vi "subVI_Strain_Ass2.vi"() -> (0 "error out":errorcluster caption="에러 출력", 3 "data 2":waveform(dbl)[](array[waveform]) caption="Strain data")   [LabVIEW 2016]
uses:
  <vilib>/DAQmx/read.llb/DAQmx Read.vi
  <vilib>/DAQmx/read.llb/DAQmx Read (Analog 1D Wfm NChan NSamp).vi
  <vilib>/DAQmx/create/channels.llb/DAQmx Create Channel (TEDS-AI-Strain-Strain Gage).vi
  <vilib>/DAQmx/create/channels.llb/DAQmx Create Channel (AI-Strain-Strain Gage).vi
  <vilib>/DAQmx/configure/timing.llb/DAQmx Timing (Sample Clock).vi
  <vilib>/DAQmx/configure/trigger.llb/DAQmx Trigger.vi
  <vilib>/DAQmx/configure/trigger.llb/DAQmx Start Trigger (Digital Edge).vi
  <vilib>/DAQmx/miscellaneous.llb/DAQmx Fill In Error Info.vi
  <resource>/objmgr/daqmx.rc
panel:
  out "task out":refnum<k21> caption="태스크 출력"
  in  "error in":errorcluster caption="에러 입력"
  out "data":dynamicdata(graph) caption="Strain"
  in  "stop (T)":bool=TRUE caption="정지(T)"
  in  "속도":dbl=50000.0
  in  "샘플 개수":i32=1000
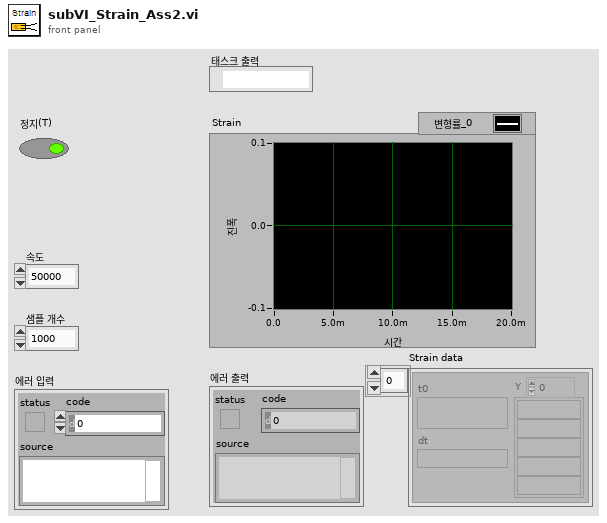
[diagram p1: front panel]
types:
  T1 = cluster{"Test Information":cluster{"date":string, "custom":string, "oper":string, "package":string, "pkg side":string, "solder":string, "brd side":string, "paste":string, "reflow":string}, "Sensor Set":cluster{"Accelerometer":cluster{"Sensitivity(mV/g)":dbl}, "Strain Guage":cluster{"Ch.":dbl[], "Gage factor":dbl[], "Resistance":dbl[], "Poisson ratio":dbl[]}}, "Resistor Set":cluster{"Criterion Level":dbl, "Res. Set":cluster{"Res. Ch":dbl, "Res. Active":bool, "Res Initial":dbl}[]}, "Test Stop Condition":cluster{"Test cycle":u16, "Fail number in a cycle":u16, "Fail factor":cluster{"Duration":u16, "Fail No.":u16}}, "Acceleration Condition ":cluster{"Shock duration pecent [%]":u16, "Filter cutoff freq":u32}, "Save":cluster{"Save Path":path, "File Name":string}}
  T2 = cluster{"Ch.":dbl[], "Gage factor":dbl[], "Resistance":dbl[], "Poisson ratio":dbl[]}
  T3 = cluster{"lead resistance":dbl, "initial bridge voltage":dbl, "excitation source":i32, "excitation value":dbl}
  T4 = cluster{"strain configuration":i32, "lead resistance":dbl, "initial bridge voltage":dbl, "excitation source":i32, "excitation value":dbl}
  T5 = cluster{"Gage factor":dbl, "Resistance":dbl, "Poisson ratio":dbl}
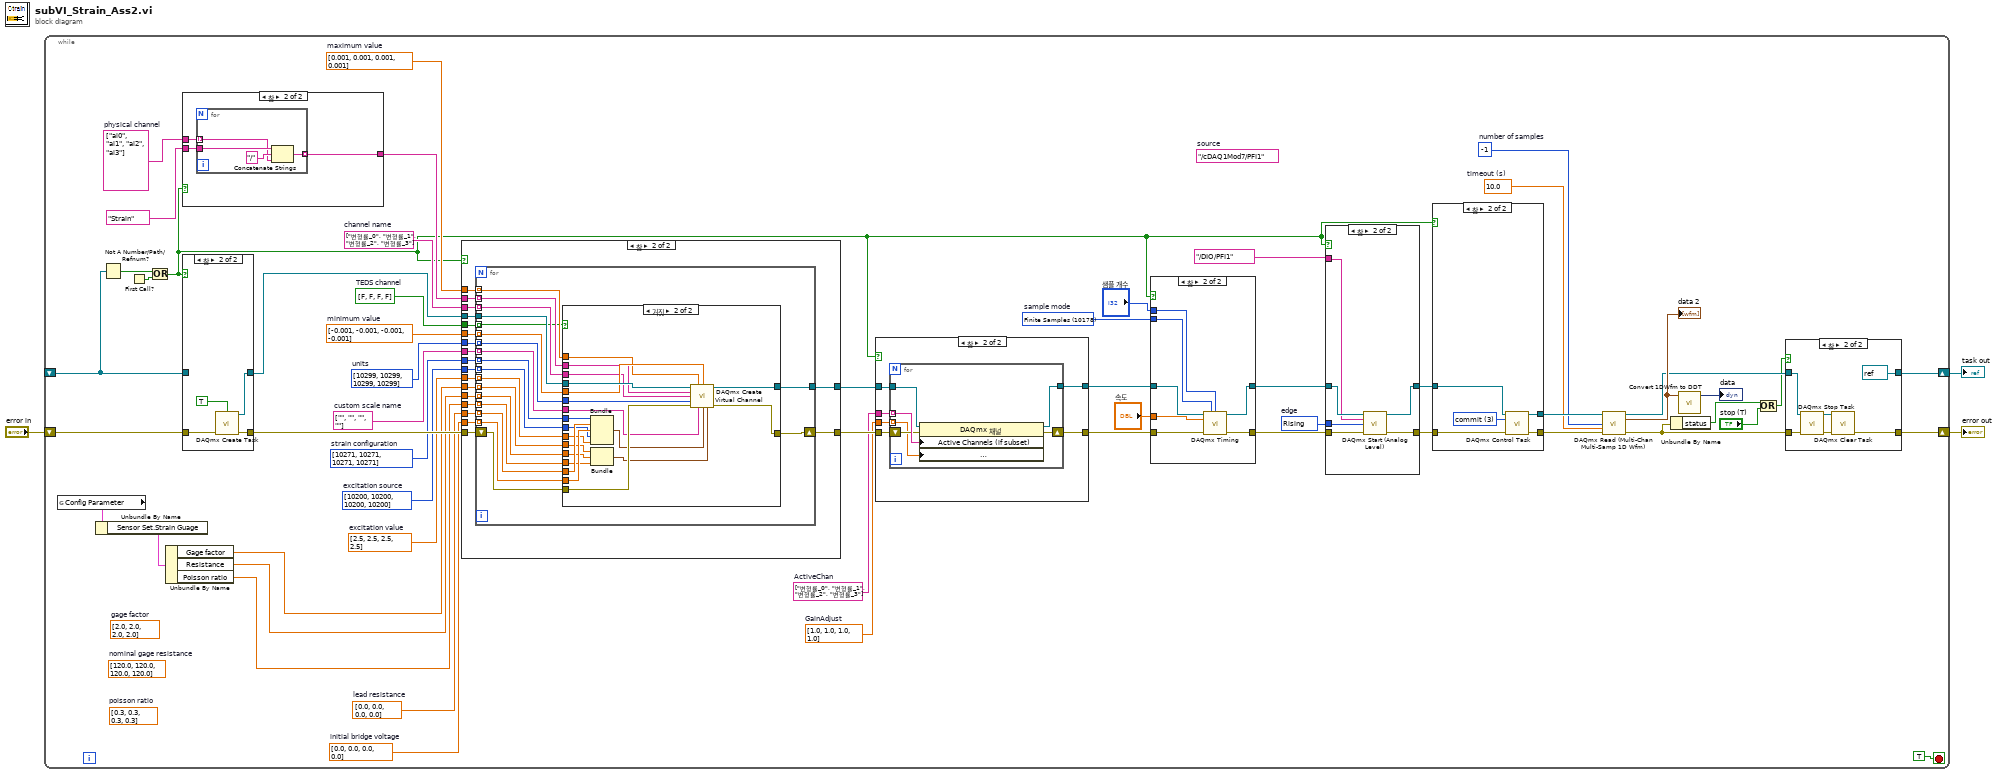
[diagram p0: block diagram]
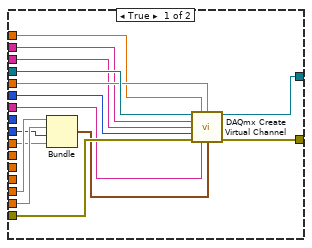
[diagram p8: hidden frame]
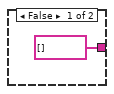
[diagram p9: hidden frame]
diagram:
  n1 = while {
    shift-right: [w16] -> w1
    shift-left: _ -> [w55]
    shift-right: [w14] -> w2
    shift-left: "error in" -> [w56]
    stop <- TRUE stop-if-true
    w18 = 10.0  # timeout (s)
    w20 = -1  # number of samples
    w26 = 10280 items=["Rising"=10280, "Falling"=10171]  # edge
    (unwired) "/cDAQ1Mod7/PFI1"  # source
    w29 = 10178 items=["Finite Samples"=10178, "Continuous Samples"=10123, "Hardware Timed Single Point"=12522]  # sample mode
    w34 = dbl[] [1.0, 1.0, 1.0, 1.0]  # GainAdjust
    w35 = string[] ["변형률_0", "변형률_1", "변형률_2", "변형률_3"]  # ActiveChan
    w38 = bool[] [FALSE, FALSE, FALSE, FALSE]  # TEDS channel
    (unwired) dbl[] [0.3, 0.3, 0.3, 0.3]  # poisson ratio
    (unwired) dbl[] [120.0, 120.0, 120.0, 120.0]  # nominal gage resistance
    (unwired) dbl[] [2.0, 2.0, 2.0, 2.0]  # gage factor
    w39 = dbl[] [2.5, 2.5, 2.5, 2.5]  # excitation value
    w40 = i32[] [10200, 10200, 10200, 10200] items=["Internal"=10200, "External"=10167, "None"=10230]  # excitation source
    w41 = dbl[] [0.0, 0.0, 0.0, 0.0]  # initial bridge voltage
    w43 = i32[] [10271, 10271, 10271, 10271] items=["Full Bridge I"=10183, "Full Bridge II"=10184, "Full Bridge III"=10185, "Half Bridge I"=10188, "Half Bridge II"=10189, "Quarter Bridge I"=10271, "Quarter Bridge II"=10272]  # strain configuration
    w42 = dbl[] [0.0, 0.0, 0.0, 0.0]  # lead resistance
    w44 = string[] ["", "", "", ""]  # custom scale name
    w45 = i32[] [10299, 10299, 10299, 10299] items=["Strain"=10299, "From Custom Scale"=10065]  # units
    w46 = string[] ["변형률_0", "변형률_1", "변형률_2", "변형률_3"]  # channel name
    w48 = dbl[] [0.001, 0.001, 0.001, 0.001]  # maximum value
    w49 = dbl[] [-0.001, -0.001, -0.001, -0.001]  # minimum value
    w52 = string[] ["ai0", "ai1", "ai2", "ai3"]  # physical channel
    n2 = global read "글로벌_Config Parameter.vi" "Config Parameter"() -> (w8:T1)
    n3 = Unbundle By Name(w8) -> ("Sensor Set.Strain Guage"=w7:T2)
    n4 = Not A Number/Path/Refnum?(number/path/refnum=w55) -> (NaN/Path/Refnum?=w54:bool)
    n5 = First Call?() -> (First Call?: T/F=w57:bool)
    n6 = Or(x=w54, y=w57) -> (x .or. y?=w25:bool)
    n7 = Unbundle By Name(w7) -> ("Gage factor"=w4:dbl[], "Resistance"=w5:dbl[], "Poisson ratio"=w6:dbl[])
    n8 = case "케이스 구조" shown="참" w25 {
      tunnel: [string[] [] w183] -> w47
      tunnel: tag "Strain" ("디바이스 이름") -> [_ w182]
      tunnel: w52 -> [_ w181]
      frame False {
      }
      frame True {
        n9 = for "For 루프" {
          tunnel: [w187] -> w183 mode=indexing
          tunnel: w182 -> [w186]
          tunnel: w181 -> [w184] mode=indexing
          n10 = Concatenate Strings(w186, "/" ("string"), w184) -> (w187:string)
        }
      }
    }
    n11 = case "케이스 구조" shown="참" w25 {
      tunnel: [w189 w193] -> w51
      tunnel: w55 -> [w189 _]
      tunnel: [w188 w192] -> w50
      tunnel: w56 -> [w188 w190]
      frame False {
      }
      frame True {
        n12 = call <vilib>:"DAQmx Create Task.vi"("auto cleanup"=TRUE, "error in"=w190) -> ("task out"=w193:refnum<k21>, "error out"=w192:errorcluster)  [unwired: 12 in]
      }
    }
    n13 = case "케이스 구조" shown="참" w25 {
      tunnel: [w106 w123] -> w37
      tunnel: w51 -> [w106 w125]
      tunnel: [w105 w122] -> w36
      tunnel: w50 -> [w105 w124]
      tunnel: w49 -> [_ w121]
      tunnel: w48 -> [_ w120]
      tunnel: w47 -> [_ w119]
      tunnel: w46 -> [_ w118]
      tunnel: w45 -> [_ w117]
      tunnel: w44 -> [_ w116]
      tunnel: w43 -> [_ w115]
      tunnel: w42 -> [_ w114]
      tunnel: w41 -> [_ w113]
      tunnel: w40 -> [_ w112]
      tunnel: w39 -> [_ w111]
      tunnel: w4 -> [_ w110]
      tunnel: w5 -> [_ w109]
      tunnel: w6 -> [_ w108]
      tunnel: w38 -> [_ w107]
      frame False {
      }
      frame True {
        n14 = for "For 루프" {
          tunnel: w125 -> [w144]
          tunnel: [w142] -> w123
          tunnel: w121 -> [w140] mode=indexing
          tunnel: w120 -> [w139] mode=indexing
          tunnel: w119 -> [w138] mode=indexing
          tunnel: w118 -> [w137] mode=indexing
          shift-right: [w141] -> w122
          shift-left: w124 -> [w143]
          tunnel: w117 -> [w136] mode=indexing
          tunnel: w116 -> [w135] mode=indexing
          tunnel: w115 -> [w134] mode=indexing
          tunnel: w114 -> [w133] mode=indexing
          tunnel: w113 -> [w132] mode=indexing
          tunnel: w112 -> [w131] mode=indexing
          tunnel: w111 -> [w130] mode=indexing
          tunnel: w110 -> [w129] mode=indexing
          tunnel: w109 -> [w128] mode=indexing
          tunnel: w108 -> [w127] mode=indexing
          tunnel: w107 -> [w126] mode=indexing
          n15 = case "케이스 구조" shown="거짓" w126 {
            tunnel: w144 -> [w159 w179]
            tunnel: w143 -> [w158 w178]
            tunnel: [w157 w177] -> w142
            tunnel: [w156 w176] -> w141
            tunnel: w140 -> [w155 w175]
            tunnel: w139 -> [w154 w174]
            tunnel: w138 -> [w153 w173]
            tunnel: w137 -> [w152 w172]
            tunnel: w136 -> [w150 w170]
            tunnel: w135 -> [w149 w169]
            tunnel: w134 -> [_ w168]
            tunnel: w133 -> [w148 w167]
            tunnel: w132 -> [w147 w166]
            tunnel: w131 -> [w146 w165]
            tunnel: w130 -> [w145 w164]
            tunnel: w129 -> [_ w163]
            tunnel: w128 -> [_ w162]
            tunnel: w127 -> [_ w161]
            frame True {
              n16 = Bundle("lead resistance"=w148, "initial bridge voltage"=w147, "excitation source"=w146, "excitation value"=w145) -> (w151:T3)  [unwired: 1 in]
              n17 = call-poly <vilib>:"DAQmx Create Virtual Channel.vi"("task in"=w159, "maximum value"=w154, "minimum value"=w155, "physical channels"=w153, "name to assign"=w152, "units"=w150, "error in"=w158, "custom scale name"=w149, "bridge information"=w151) -> ("task out"=w157:refnum<k21>, "error out"=w156:errorcluster)  [unwired: 5 in]
            }
            frame False {
              n18 = Bundle("strain configuration"=w168, "lead resistance"=w167, "initial bridge voltage"=w166, "excitation source"=w165, "excitation value"=w164) -> (w171:T4)  [unwired: 1 in]
              n19 = Bundle("Gage factor"=w163, "Resistance"=w162, "Poisson ratio"=w161) -> (w160:T5)  [unwired: 1 in]
              n20 = call-poly <vilib>:"DAQmx Create Virtual Channel.vi"("task in"=w179, "maximum value"=w174, "minimum value"=w175, "physical channels"=w173, "name to assign"=w172, "units"=w170, "error in"=w178, "custom scale name"=w169, "bridge information"=w171, "strain gage information"=w160) -> ("task out"=w177:refnum<k21>, "error out"=w176:errorcluster)  [unwired: 4 in]
            }
          }
        }
      }
    }
    n21 = case "케이스 구조" shown="참" w25 {
      tunnel: [w92 w95] -> w33
      tunnel: w37 -> [w92 w98]
      tunnel: [w91 w96] -> w32
      tunnel: w36 -> [w91 w97]
      tunnel: w35 -> [_ w94]
      tunnel: w34 -> [_ w93]
      frame False {
      }
      frame True {
        n22 = for "For 루프" {
          tunnel: w98 -> [w104]
          shift-right: [w102] -> w96
          shift-left: w97 -> [w100]
          tunnel: [w103] -> w95
          tunnel: w94 -> [w101] mode=indexing
          tunnel: w93 -> [w99] mode=indexing
          n23 = property class="DAQmx 채널"(reference=w104, error in=w100, "Active Channels (if subset)"=w101, "Analog Input:General Properties:Signal Conditioning:Bridge:Shunt Cal:Gain Adjustment"=w99) -> (reference out=w103:refnum<k21>, error out=w102:errorcluster)
        }
      }
    }
    n24 = case "케이스 구조" shown="참" w25 {
      tunnel: [w83 w85] -> w28
      tunnel: w33 -> [w83 w88]
      tunnel: [w82 w84] -> w27
      tunnel: w32 -> [w82 w86]
      tunnel: "샘플 개수" -> [_ w90]
      tunnel: w29 -> [_ w89]
      tunnel: "속도" -> [_ w87]
      frame False {
      }
      frame True {
        n25 = call-poly <vilib>:"DAQmx Timing.vi"("task/channels in"=w88, "sample mode"=w89, "samples per channel"=w90, "rate"=w87, "error in"=w86) -> ("task out"=w85:refnum<k21>, "error out"=w84:errorcluster)  [unwired: 9 in]
      }
    }
    n26 = case "케이스 구조" shown="참" w25 {
      tunnel: [w75 w79] -> w24
      tunnel: w28 -> [w75 w81]
      tunnel: [w74 w78] -> w23
      tunnel: w27 -> [w74 w80]
      tunnel: tag "/DIO/PFI1" ("source") -> [_ w77]
      tunnel: w26 -> [_ w76]
      frame False {
      }
      frame True {
        n27 = call-poly "DAQmx Start (Analog Level).vi"("task/channels in"=w81, "source"=w77, "edge"=w76, "error in"=w80) -> ("task out"=w79:refnum<k21>, "error out"=w78:errorcluster)  [unwired: 10 in]
      }
    }
    n28 = case "케이스 구조" shown="참" w25 {
      tunnel: [w68 w72] -> w22
      tunnel: w24 -> [w68 w73]
      tunnel: [w67 w70] -> w21
      tunnel: w23 -> [w67 w71]
      frame False {
      }
      frame True {
        w69 = 3 items=["verify"=2, "reserve"=4, "commit"=3, "unreserve"=5, "abort"=6] ("action")
        n29 = call <vilib>:"DAQmx Control Task.vi"("task/channels in"=w73, "action"=w69, "error in"=w71) -> ("task out"=w72:refnum<k21>, "error out"=w70:errorcluster)  [unwired: 11 in]
      }
    }
    n30 = call-poly "DAQmx Read (Multi-Chan Multi-Samp 1D Wfm).vi"("task/channels in"=w22, "number of samples per channel"=w20, "timeout"=w18, "error in"=w21) -> ("task out"=w15:refnum<k21>, "data"=w19:waveform(dbl)[], "error out"=w13:errorcluster)  [unwired: 9 in]
    "data 2" <- w19
    n31 = Unbundle By Name(w13) -> ("status"=w12:bool)
    n32 = call <vilib>:"Convert 1DWfm to DDT.vi"("Array of Waveforms"=w19) -> ("Dynamic Data Type"=→"data":dynamicdata)  [unwired: 3 in]
    n33 = Or(x=w12, y="stop (T)") -> (x .or. y?=w10:bool)
    n34 = case "케이스 구조" shown="참" w10 {
      tunnel: [w60 refnum<k21> refnum ("task in")] -> w16
      tunnel: w15 -> [w60 w66]
      tunnel: [w59 w63] -> w14
      tunnel: w13 -> [w59 w65]
      frame False {
      }
      frame True {
        n35 = call <vilib>:"DAQmx Stop Task.vi"("task/channels in"=w66, "error in"=w65) -> ("task out"=w62:refnum<k21>, "error out"=w64:errorcluster)  [unwired: 12 in]
        n36 = call <vilib>:"DAQmx Clear Task.vi"("task in"=w62, "error in"=w64) -> ("error out"=w63:errorcluster)  [unwired: 13 in]
      }
    }
  }
  "error out" <- w2
  "task out" <- w1
